vi "Utility_GenerateTrajectory.vi"(7 "method":i32(ring)=3 items=["nearest", "linear", "spline", "cubic Hermite"], 9 "ntimes":i32=5, 11 "path":cluster{"X":sgl, "Y":sgl}[](array[cluster])=[{"X"=-2.0, "Y"=-2.0}, {"X"=-2.0, "Y"=-1.5}, {"X"=-2.0, "Y"=-1.0}, {"X"=-2.0, "Y"=-0.5}, {"X"=-2.0, "Y"=0.0}, {"X"=-2.0, "Y"=0.5}, {"X"=-1.7, "Y"=0.9}, {"X"=-1.3, "Y"=1.2}, {"X"=-0.8, "Y"=1.2}, {"X"=-0.4, "Y"=1.5}, {"X"=-0.1, "Y"=1.9}, {"X"=0.2, "Y"=2.3}, {"X"=0.5, "Y"=2.7}, {"X"=0.9, "Y"=3.0}, {"X"=1.4, "Y"=3.0}, {"X"=1.9, "Y"=3.0}, {"X"=2.3, "Y"=3.3}, {"X"=2.8, "Y"=3.3}, {"X"=3.2, "Y"=3.0}, {"X"=3.2, "Y"=2.5}, {"X"=3.2, "Y"=2.0}, {"X"=2.9, "Y"=1.6}, {"X"=2.5, "Y"=1.3}, {"X"=2.2, "Y"=0.9}, {"X"=1.9, "Y"=0.5}, {"X"=1.6, "Y"=0.1}, {"X"=1.3, "Y"=-0.3}, {"X"=1.3, "Y"=-0.8}, {"X"=1.3, "Y"=-1.3}, {"X"=1.6, "Y"=-1.7}, {"X"=2.0, "Y"=-2.0}, {"X"=2.5, "Y"=-2.0}, {"X"=2.9, "Y"=-1.7}]) -> (3 "trajectory":T1)   [LabVIEW 2017]
doc: "This VI interpolates between positions in a <b>Path</b> made up of (x, y) positions."
uses:
  Trajectory.ctl
  <vilib>/gmath/NI_Gmath.lvlib
panel:
  out "Path Graph":cluster{"yi":dbl[], "yi":dbl[]}[](graph)
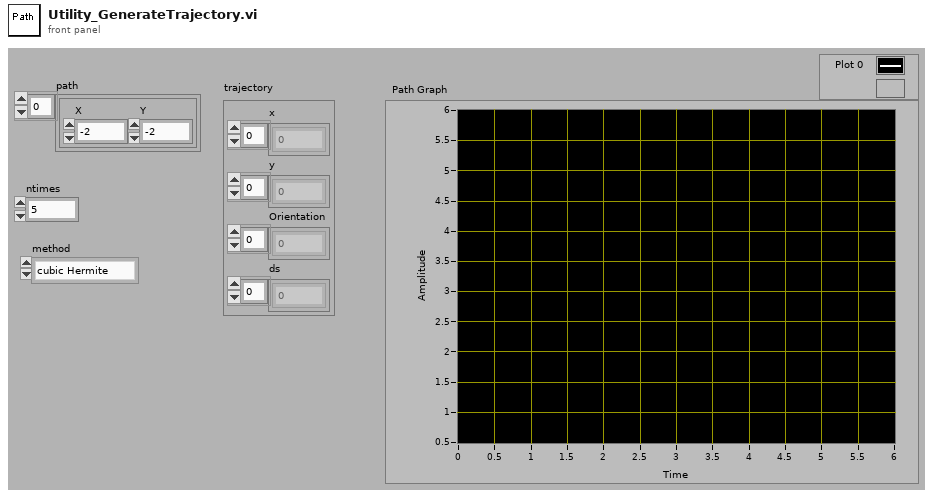
[diagram p1: front panel]
types:
  T1 = typedef "Trajectory.ctl" = cluster{"x":dbl[], "y":dbl[], "Orientation":dbl[], "ds":dbl[]}
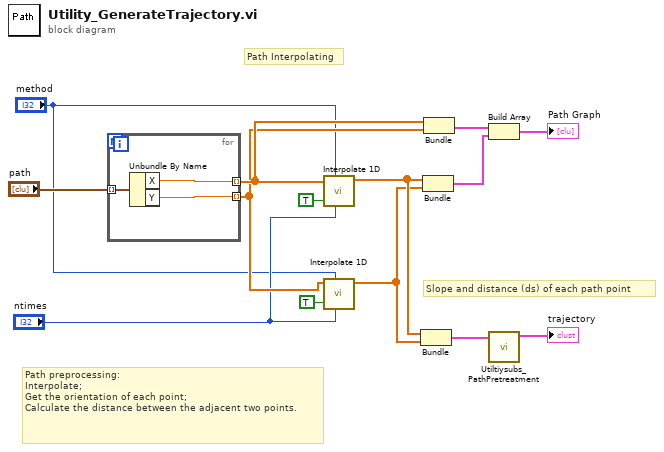
[diagram p0: block diagram]
diagram:
  # "Path preprocessing: \nInterpolate;\nGet the orientation of each point;\nCalculate the distance between the adjacent two points."
  # "Slope and distance (ds) of each path point"
  # "Path Interpolating"
  n1 = for {
    tunnel: "path" -> [w17] mode=indexing
    tunnel: [w16] -> w11 mode=indexing
    tunnel: [w15] -> w10 mode=indexing
    n2 = Unbundle By Name(w17) -> ("X"=w16:sgl, "Y"=w15:sgl)
  }
  n3 = call <vilib>:"Interpolate 1D.vi"("ntimes"="ntimes", "method"="method", "X is monotonic"=TRUE, "Y"=w11) -> ("yi"=w6:dbl[])  [unwired: 5 in, 2 out]
  n4 = call <vilib>:"Interpolate 1D.vi"("ntimes"="ntimes", "method"="method", "X is monotonic"=TRUE, "Y"=w10) -> ("yi"=w5:dbl[])  [unwired: 5 in, 2 out]
  n5 = Bundle("yi"=w6, "yi"=w5) -> (w4:cluster{"yi":dbl[], "yi":dbl[]})  [unwired: 1 in]
  n6 = Bundle("yi"=w6, "yi"=w5) -> (w8:cluster{"yi":dbl[], "yi":dbl[]})  [unwired: 1 in]
  n7 = Bundle(w11, w10) -> (w9:cluster{sgl[], sgl[]})  [unwired: 1 in]
  n8 = Build Array(w9, w8) -> (→"Path Graph":cluster{"yi":dbl[], "yi":dbl[]}[])
  n9 = call "Utiltiysubs_PathPretreatment.vi"("original trajectory"=w4) -> ("trajectory"=→"trajectory":T1)  [unwired: 10 in]
